vi "Experiment_pump_for_FR.vi"() -> ()   [LabVIEW 2016]
uses:
  <vilib>/Modbus/master/Create Master Instance (Serial).vi
  <vilib>/addons/control/pid/pid.llb/PID (DBL).vi
  <vilib>/Modbus/master/Modbus Master.lvclass
  database/database.lvlib
  <vilib>/Analysis/Matrix/NI_Matrix.lvlib
  <vilib>/addons/control/pid/NI_PID_pid.lvlib
  <vilib>/Analysis/Matrix/Numeric/Conversions/Array To Matrix - RA2.vi
panel:
  in  "单次时延(ms)":dbl
  in  "最大倍数":dbl
  out "阶跃测试输出":dbl
  out "倍数":dbl
  in  "TestId":string
  out "10s Timer":bool caption="结束"
  out "1s Timer":bool caption="结束"
  out "10ms Timer":bool caption="结束"
  in  "送风温度-流量":T1={"proportional gain (Kc)"=1.0, "integral time (Ti, min)"=40.0, "derivative time (Td, min)"=0.0}
  in  "设定流量":dbl format="%#.3f"
  in  "设定流量控制阀门-流量计读取":T1={"proportional gain (Kc)"=1.0, "integral time (Ti, min)"=40.0, "derivative time (Td, min)"=0.0}
  in  "Ctrl Strategy":u16
  in  "送风温度设定值":dbl format="%.2f"
  out "自动设定出风温度":dbl format="%.2f"
  in  "室内温度控制送风温度":T1={"proportional gain (Kc)"=1.0, "integral time (Ti, min)"=40.0, "derivative time (Td, min)"=0.0}
  in  "T setpoint":dbl format="%.2f"
  in  "根据阀门控制频率":T1={"proportional gain (Kc)"=1.0, "integral time (Ti, min)"=40.0, "derivative time (Td, min)"=0.0}
  in  "阀门开度设定值":dbl format="%.2f"
  in  "送风温度控制阀门":T1={"proportional gain (Kc)"=1.0, "integral time (Ti, min)"=40.0, "derivative time (Td, min)"=0.0}
  in  "电力控制水泵频率":T1={"proportional gain (Kc)"=1.0, "integral time (Ti, min)"=40.0, "derivative time (Td, min)"=0.0}
  in  "温差设定值":dbl format="%.2f"
  out "标记":dbl
  out "送回风温差":dbl
  in  "旁通压差设定值":dbl format="%.2f"
  out "阀门设定开度":dbl format="%.2f"
  in  "PID gains 2":T1={"proportional gain (Kc)"=1.0, "integral time (Ti, min)"=40.0, "derivative time (Td, min)"=0.0}
  in  "PID gains":T1={"proportional gain (Kc)"=1.0, "integral time (Ti, min)"=40.0, "derivative time (Td, min)"=0.0}
  in  "手动水泵频率设定":u16
  out "循环次数":i32
  out "水泵电耗设定值":dbl
  out "Data 2":string[][](array[string])
  in  "错误输入 16":errorcluster caption="错误输入"
  out "进水温度":sgl format="%.1f"
  out "频率":dbl caption="频  率" format="%.2f"
  out "error out 3":errorcluster
  in  "error in (no error)":errorcluster
  out "error out 2":errorcluster
  out "Data":string[][](array[string])
  out "布尔":bool
  in  "时间选择":bool
  out "波形图表":dynamicdata(graph)
  in  "手动加热百分比":u16 step=1
  out "error out 9":errorcluster
  in  "按时间查询":bool
  in  "多列列表框":i32(listbox)
  out "错误输出":errorcluster
  out "水泵转速":sgl format="%.2f"
  in  "出水温度设定":dbl step=1.0
  out "加热百分比":sgl format="%.2f"
  out "pv测量值":u16[](array[numeric]) caption="寄存器值"
  in  "阀设定开度":u16 step=1
  out "水泵设定频率":dbl step=1.0
  in  "error in (no error) 8":errorcluster caption="错误输入（无错误）"
  out "error out 6":errorcluster caption="错误输出"
  out "流量":dbl format="%.2f"
  out "进出口压力":dbl caption="进出口压差" format="%.2f"
  out "支管压差":dbl format="%.2f"
  out "回水温度":dbl format="%.1f"
  out "送风温度":dbl format="%.1f"
  out "回风温度":dbl format="%.1f"
  out "阀门开度":dbl format="%.2f"
  out "模拟量采集模块BD4141E 2":u16[](array[numeric]) caption="寄存器值"
  in  "error in (no error) 7":errorcluster caption="错误输入（无错误）"
  out "error out 5":errorcluster caption="错误输出"
  out "电流":dbl format="%#_4f"
  out "电压":dbl format="%.2f"
  out "水泵功率":dbl format="%.2f"
  in  "error in (no error) 3":errorcluster caption="错误输入（无错误）"
  out "通讯状态":bool
  in  "Stop":bool
  # "设  备   的  名  字"
  # "阶跃信号控制"
  # "设备的"
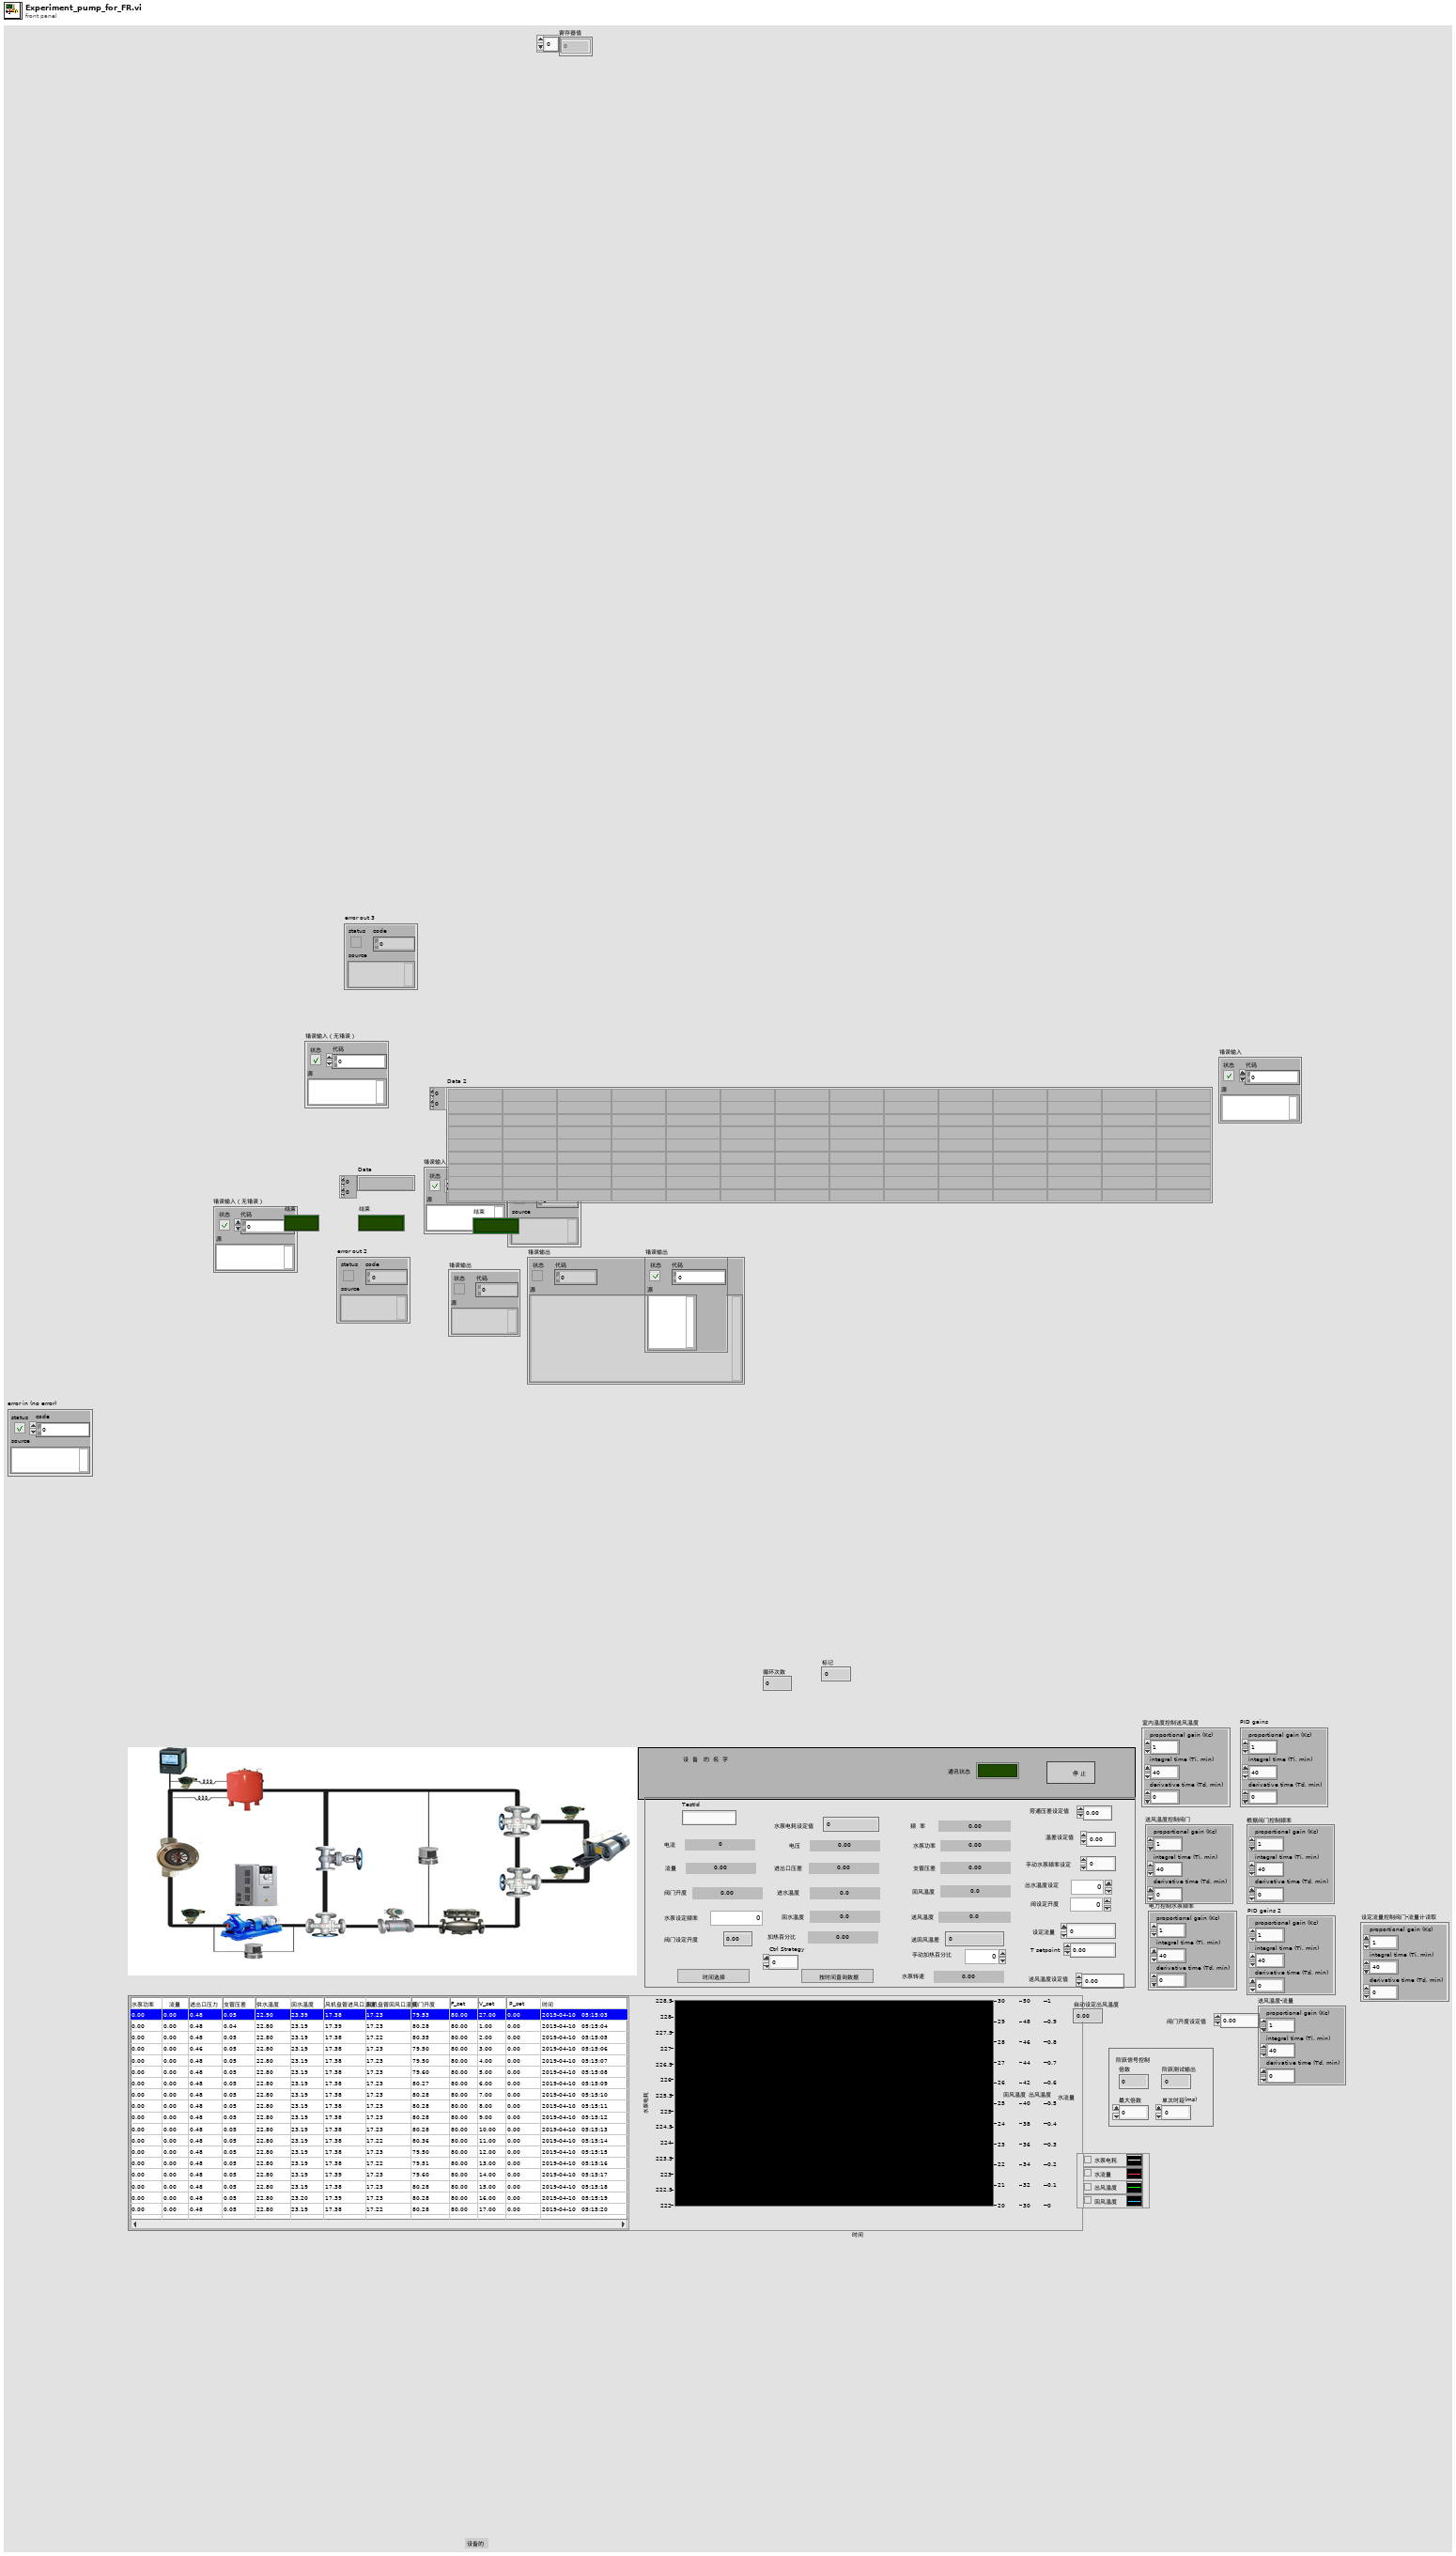
[diagram p1: front panel]
types:
  T1 = cluster{"proportional gain (Kc)":dbl, "integral time (Ti, min)":dbl, "derivative time (Td, min)":dbl}
  T2 = typedef "NI_Matrix.lvlib/RealMatrix.ctl" = dbl[][]
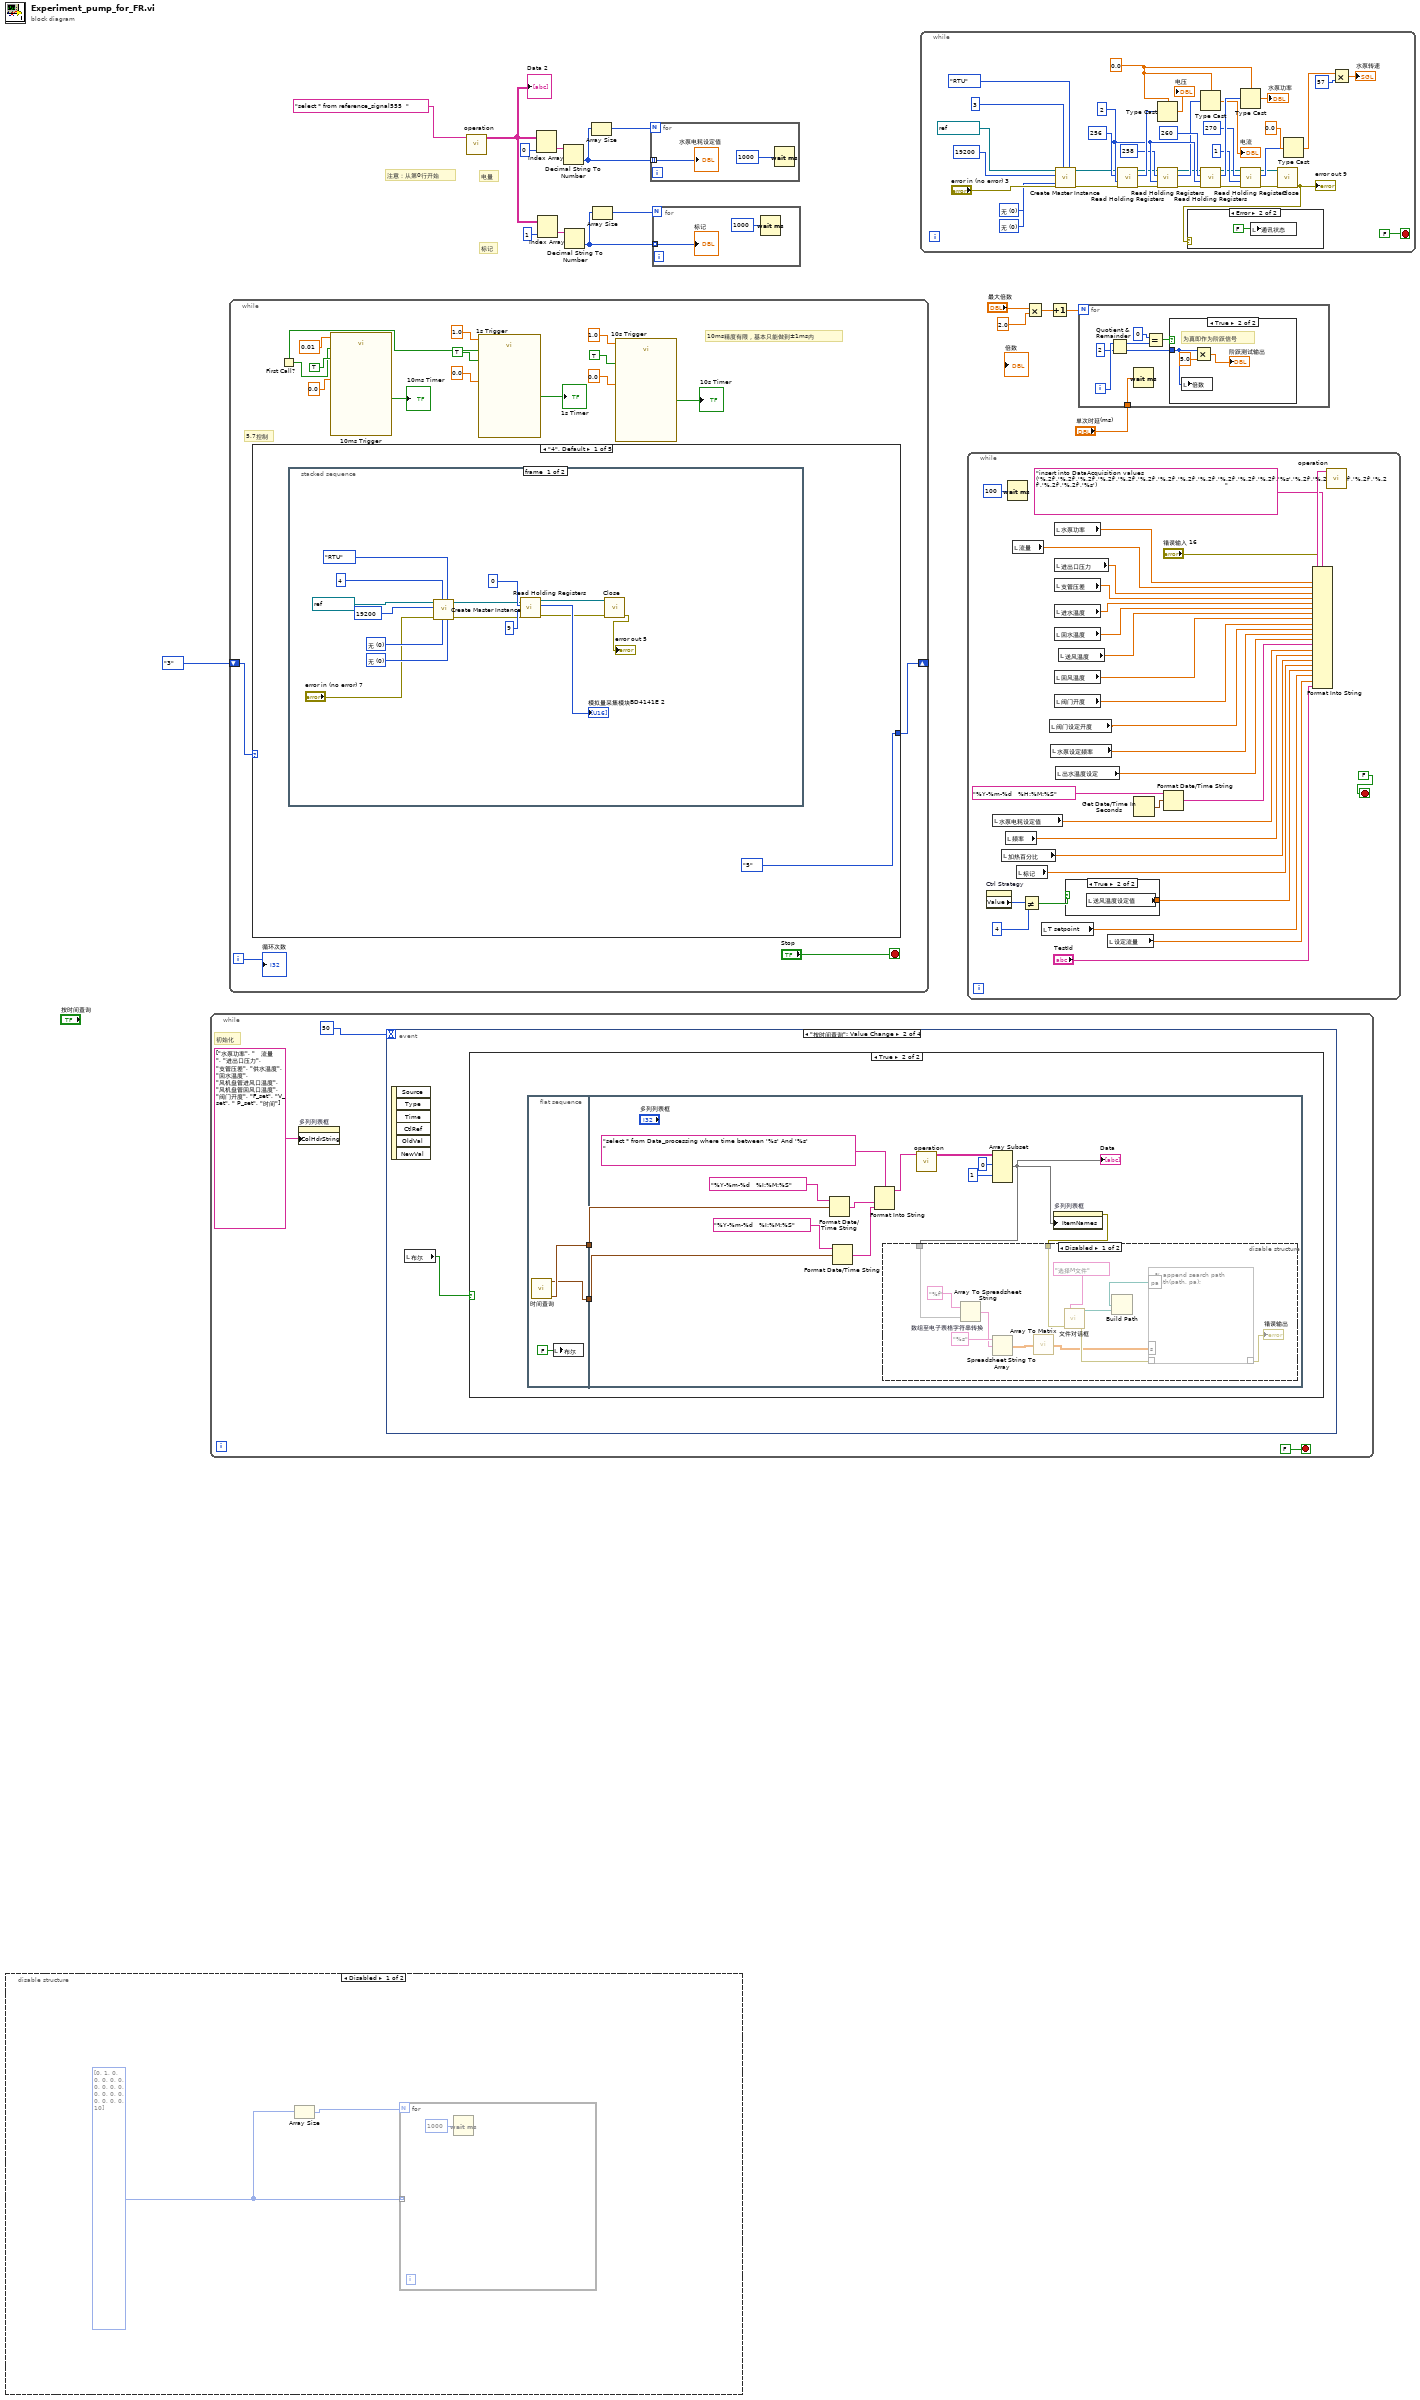
[diagram p0: block diagram]
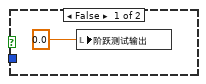
[diagram p2: hidden frame]
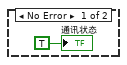
[diagram p3: hidden frame]
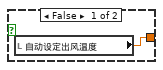
[diagram p4: hidden frame]
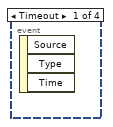
[diagram p6: hidden frame]
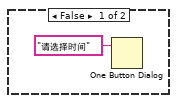
[diagram p7: hidden frame]
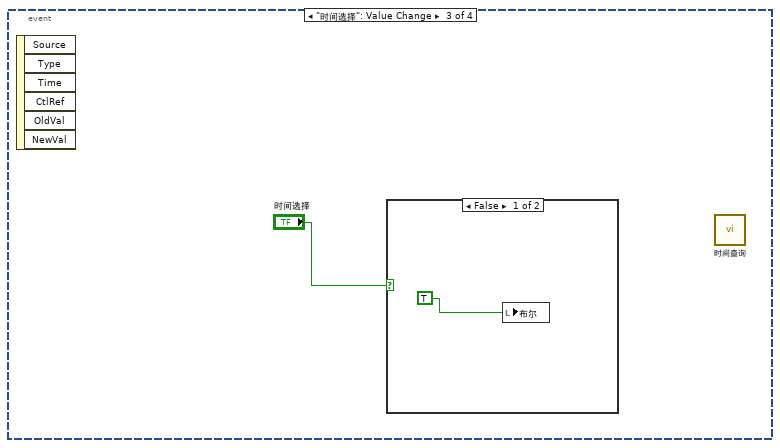
[diagram p9: hidden frame]
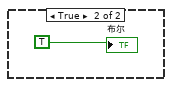
[diagram p10: hidden frame]
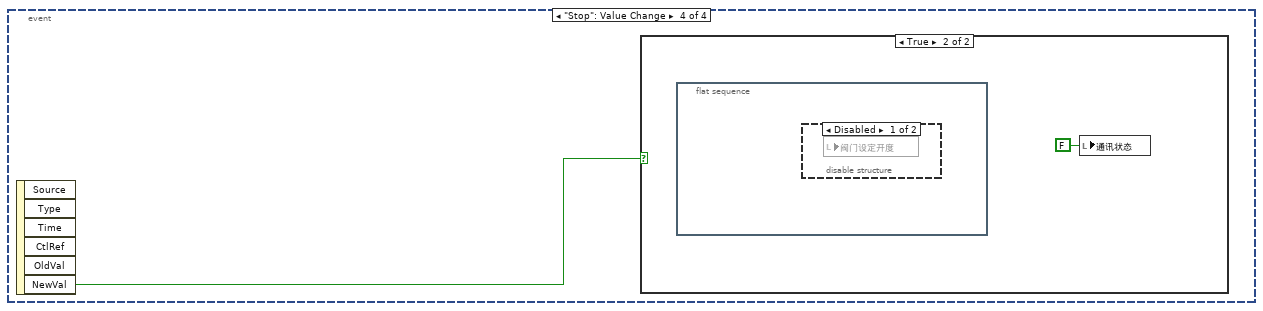
[diagram p11: hidden frame]
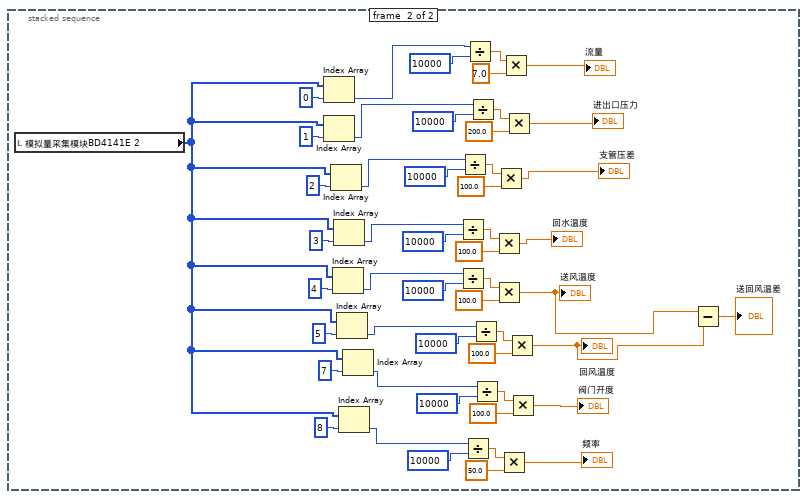
[diagram p14: hidden frame]
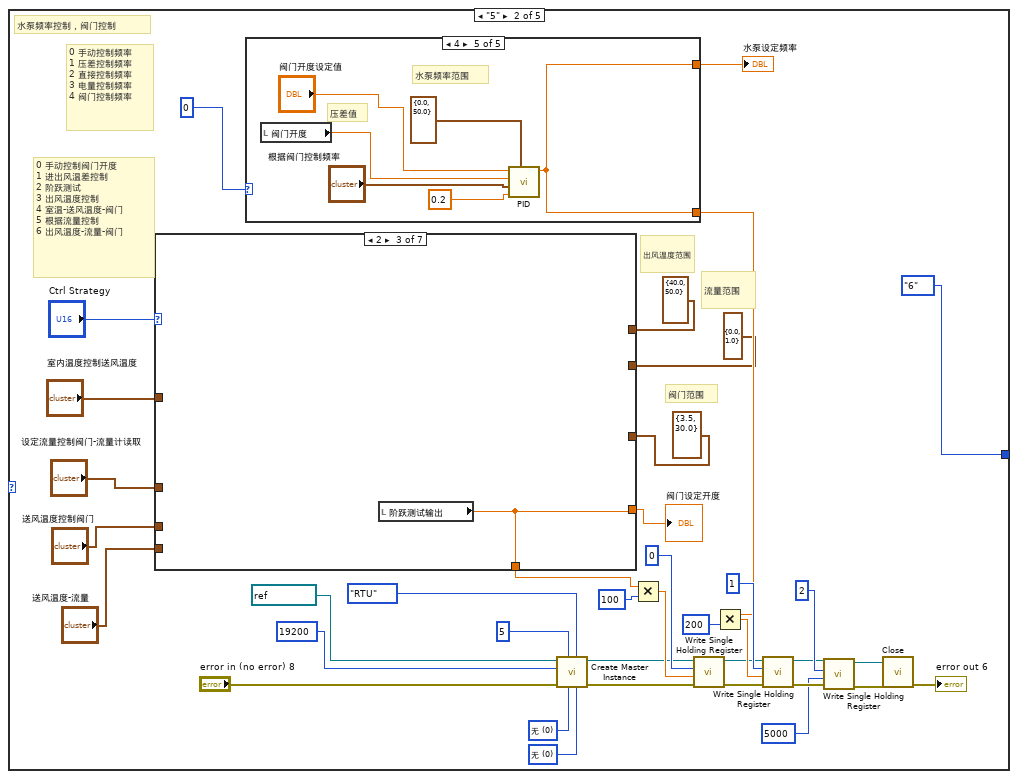
[diagram p15: hidden frame]
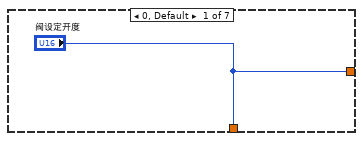
[diagram p16: hidden frame]
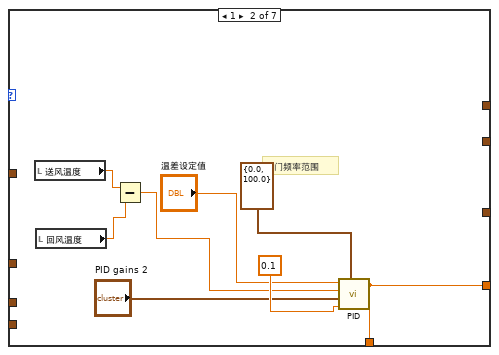
[diagram p17: hidden frame]
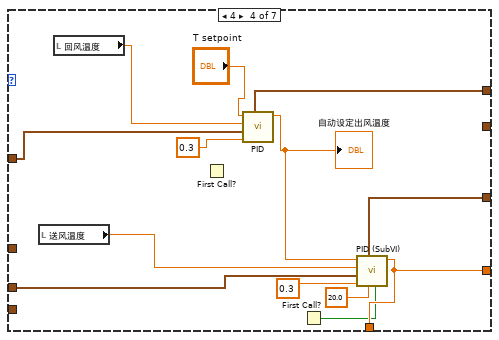
[diagram p18: hidden frame]
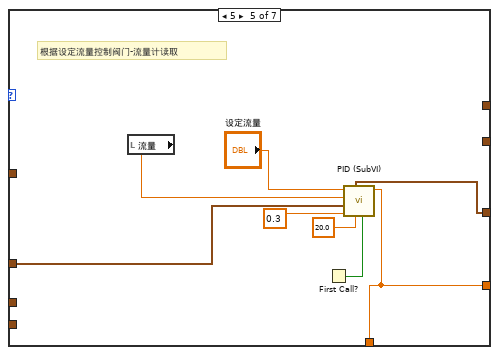
[diagram p19: hidden frame]
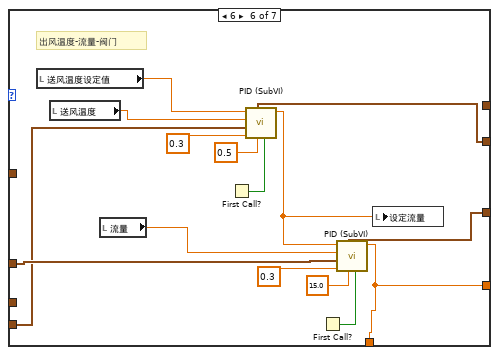
[diagram p20: hidden frame]
diagram:
  # "注意：从第0行开始"
  # "电量"
  # "标记"
  n1 = disable-structure shown="Disabled" {
    frame Disabled {
      w18 = i32[] [0, 1, 0, 0, 0, 0, 0, 0, 0, 0, 0, 0, 0, 0, 0, 0, 0, 0, 0, 10]
      n2 = Array Size(array=w18) -> (size(s)=w17:i32)
      n3 = for {
        N: w17 -> [_]
        tunnel: w18 -> [_] mode=indexing
        n4 = Wait (ms)(milliseconds to wait=u32 1000) -> ()  [unwired: 1 out]
      }
    }
    frame Enabled {
    }
  }
  n5 = while {
    stop <- FALSE stop-if-true
    # "初始化"
    n6 = property on="多列列表框" class="MCListbox (strict)"("ColHdrString"=string[] ["水泵功率", "   流量               ", "进出口压力", "支管压差", "供水温度", "回水温度", "风机盘管进风口温度", "风机盘管回风口温度", "阀门开度", "F_set", "V_set", " P_set", "时间"]) -> ()  [unwired: 2 in, 2 out]
    n7 = event shown="[1] \"按时间查询\": Value Change" {
      selector: _ -> [_ _ _ _]
      dyn-events: _ -> [_ _ _ _]
      timeout: 50 -> [_ _ _ _]
      event Timeout {
        n8 = event-data() -> ()  [unwired: 1 in, 3 out]
      }
      event "按时间查询": Value Change {
        n9 = event-data() -> ()  [unwired: 1 in, 6 out]
        n10 = local read "布尔"() -> (w23:bool)
        n11 = case shown="True" w23 {
          frame False {
            n12 = One Button Dialog(message="请选择时间" ("消息")) -> ()  [unwired: 1 in, 1 out]
          }
          frame True {
            n13 = flat-sequence {
              tunnel: [w28] -> w26
              tunnel: [w27] -> w25
              tunnel: w26 -> [w36]
              tunnel: w25 -> [w35]
              frame #0 {
                n14 = call "时间查询.vi"() -> ("时间标识 3"=w28:timestamp, "时间标识 4"=w27:timestamp)  [unwired: 8 in]
                n15 = local write "布尔"(FALSE ("布尔")) -> ()
              }
              frame #1 {
                n16 = Format Date/Time String(time format string (%c)="%Y-%m-%d   %I:%M:%S" ("时间格式字符串(%c)"), seconds (now)=w36) -> (date/time string=w40:string)  [unwired: 1 in]
                n17 = Format Date/Time String(time format string (%c)="%Y-%m-%d   %I:%M:%S" ("时间格式字符串(%c)"), seconds (now)=w35) -> (date/time string=w42:string)  [unwired: 1 in]
                n18 = Format Into String(format string="select * from Data_processing where time between '%s' And '%s'                                                                " ("格式字符串"), w40, w42) -> (resulting string=w37:string)  [unwired: 2 in, 1 out]
                n19 = call "operation.vi"("Command Text"=w37) -> ("Data"=w33:string[][])  [unwired: 9 in]
                n20 = Array Subset(array=w33, index (row)=0 ("index"), index (col)=1 ("index")) -> (w30:string[][])  [unwired: 2 in]
                "Data" <- w30
                n21 = property on="多列列表框" class="MCListbox (strict)"("ItemNames"=w30) -> (error out=w34:errorcluster)  [unwired: 2 in, 1 out]
                n22 = disable-structure shown="Disabled" {
                  disable-tunnel: w34 -> [w54 _]
                  disable-tunnel: w30 -> [w53 _]
                  frame Disabled {
                    n23 = Array To Spreadsheet String "数组至电子表格字符串转换"(array=w53, 3:"%f" ("格式字符串")) -> (spreadsheet string=w49:string)  [unwired: 1 in]
                    n24 = Spreadsheet String To Array(format string="%s" ("格式字符串"), spreadsheet string=w49) -> (array=w50:dbl[][])  [unwired: 2 in]
                    n25 = call-poly <vilib>:"Array To Matrix.vi"("Real 2D Array"=w50) -> ("Real Matrix"=w44:T2)
                    n26 = call "文件对话框"("prompt"="选择M文件", "error in"=w54) -> ("selected path"=w47:path, "error out"=w45:errorcluster)  [unwired: 10 in, 2 out]
                    n27 = Build Path(name or relative path=w47) -> (appended path=w46:path)  [unwired: 1 in]
                    n28 = script code="% append search path\npath(path, pa);"("??"=w45, "pa"=w46, "s"=w44) -> ("??"=→"错误输出":errorcluster)
                  }
                  frame Enabled {
                  }
                }
              }
            }
          }
        }
      }
      event "时间选择": Value Change {
        n29 = event-data() -> ()  [unwired: 1 in, 6 out]
        n30 = case shown="False" "时间选择" {
          frame False {
            n31 = local write "布尔"(TRUE) -> ()
          }
          frame True {
            "布尔" <- TRUE
          }
        }
        n32 = call "时间查询.vi"() -> ()  [unwired: 8 in, 2 out]
      }
      event "Stop": Value Change {
        n33 = event-data() -> ("NewVal"=w58:bool)  [unwired: 1 in, 5 out]
        n34 = case shown="True" w58 {
          frame False {
          }
          frame True {
            n35 = flat-sequence {
              frame #0 {
                n36 = disable-structure shown="Disabled" {
                  frame Disabled {
                    n37 = local read "阀门设定开度"() -> ()  [unwired: 1 in]
                  }
                  frame Enabled {
                  }
                }
              }
            }
            n38 = local write "通讯状态"(FALSE ("通讯状态")) -> ()
          }
        }
      }
    }
  }
  n39 = while {
    shift-right: [w75] -> _
    shift-left: enum16{"3", "4", "5", "6", "7", "8", "9", "10"}."3" -> [w76]
    i -> [w73]
    stop <- "Stop" stop-if-true
    # "10ms精度有限，基本只能做到±1ms内"
    # "5,7控制"
    n40 = case shown="\"4\", Default" w76 {
      tunnel: [enum16{"3", "4", "5", "6", "7", "8", "9", "10"}."5" enum16{"3", "4", "5", "6", "7", "8", "9", "10"}."6" enum16{"3", "4", "5", "6", "7", "8", "9", "10"}."7" enum16{"3", "4", "5", "6", "7", "8", "9", "10"}."8" enum16{"3", "4", "5", "6", "7", "8", "9", "10"}."3"] -> w75
      frame "4", Default {
        n41 = stacked-sequence {
          frame #0 {
            w86 = u16 0 items=["无", "XON/XOFF", "RTS/CTS", "XON/XOFF & RTS/CTS", "DTR/DSR", "XON/XOFF & DTR/DSR"] ("flow control (None)")
            w87 = u16 0 items=["无", "奇", "偶"] ("parity (Even)")
            n42 = call-poly <vilib>:"Create Master Instance.vi"("flow control (None)"=w86, "serial type"=enum16{"RTU", "ASCII"}."RTU", "parity (Even)"=w87, "unit ID"=u8 4, "error in (no error)"="error in (no error) 7", "baud rate (9600)"=u32 19200, "VISA resource name"=refnum<visa-resource-name> "COM4") -> ("error out"=w82:errorcluster, "serial master instance"=w79:refnum<class "Modbus Master.lvclass">)  [unwired: 3 in]
            n43 = call-dynamic "Read Holding Registers.vi"("error in (no error)"=w82, "number of holding registers"=u16 9, "starting address"=u16 0, "Modbus master in"=w79) -> ("error out"=w81:errorcluster, "register values"=→"模拟量采集模块BD4141E 2":u16[], "Modbus master out"=w78:refnum<class "Modbus Master.lvclass">)  [unwired: 5 in]
            n44 = call-dynamic "Close.vi"("error in (no error)"=w81, "Modbus master in"=w78) -> ("error out"=→"error out 5":errorcluster)  [unwired: 9 in]
          }
          frame #1 {
            n45 = local read "模拟量采集模块BD4141E 2"() -> (w102:u16[])
            n46 = Index Array(array=w102, index=0 ("索引")) -> (element=w135:u16)
            n47 = Index Array(array=w102, index=1 ("索引")) -> (element=w129:u16)
            n48 = Index Array(array=w102, index=2 ("索引")) -> (element=w123:u16)
            n49 = Index Array(array=w102, index=4 ("索引")) -> (element=w113:u16)
            n50 = Index Array(array=w102, index=3 ("索引")) -> (element=w119:u16)
            n51 = Index Array(array=w102, index=5 ("索引")) -> (element=w109:u16)
            n52 = Index Array(array=w102, index=8 ("索引")) -> (element=w98:u16)
            n53 = Index Array(array=w102, index=7 ("索引")) -> (element=w106:u16)
            n54 = Divide(x=w119, y=u16 10000) -> (x/y=w114:dbl)
            n55 = Divide(x=w113, y=u16 10000) -> (x/y=w115:dbl)
            n56 = Divide(x=w123, y=u16 10000) -> (x/y=w126:dbl)
            n57 = Divide(x=w98, y=u16 10000) -> (x/y=w101:dbl)
            n58 = Divide(x=w135, y=u16 10000) -> (x/y=w133:dbl)
            n59 = Divide(x=w129, y=u16 10000) -> (x/y=w128:dbl)
            n60 = Divide(x=w109, y=u16 10000) -> (x/y=w112:dbl)
            n61 = Divide(x=w106, y=u16 10000) -> (x/y=w105:dbl)
            n62 = Multiply(x=w114, y=100.0) -> (x*y=→"回水温度":dbl)
            n63 = Multiply(x=w115, y=100.0) -> (x*y=w96:dbl)
            "送风温度" <- w96
            n64 = Multiply(x=w126, y=100.0) -> (x*y=→"支管压差":dbl)
            n65 = Multiply(x=w101, y=50.0) -> (x*y=→"频率":dbl)
            n66 = Multiply(x=w133, y=7.0) -> (x*y=→"流量":dbl)
            n67 = Multiply(x=w128, y=200.0) -> (x*y=→"进出口压力":dbl)
            n68 = Multiply(x=w112, y=100.0) -> (x*y=w95:dbl)
            "回风温度" <- w95
            n69 = Multiply(x=w105, y=100.0) -> (x*y=→"阀门开度":dbl)
            n70 = Subtract(x=w96, y=w95) -> (x-y=→"送回风温差":dbl)
          }
        }
      }
      frame "5" {
        w174 = u16 0 items=["无", "XON/XOFF", "RTS/CTS", "XON/XOFF & RTS/CTS", "DTR/DSR", "XON/XOFF & DTR/DSR"] ("flow control (None)")
        w176 = u16 0 items=["无", "奇", "偶"] ("parity (Even)")
        # "流量范围"
        # "出风温度范围"
        # "阀门范围"
        # "0 手动控制阀门开度\n1 进出风温差控制\n2 阶跃测试\n3 出风温度控制\n4 室温-送风温度-阀门\n5 根据流量控制\n6 出风温度-流量-阀门"
        # "0 手动控制频率\n1 压差控制频率\n2 直接控制频率\n3 电量控制频率\n4 阀门控制频率"
        # "水泵频率控制，阀门控制"
        n71 = case shown="2" "Ctrl Strategy" {
          tunnel: ["阀设定开度" w182 w190 w200 w208 w223 w232] -> w161
          tunnel: ["阀设定开度" w182 w190 w200 w208 w223 w232] -> w160
          tunnel: "设定流量控制阀门-流量计读取" -> [_ _ _ _ w207 w221 _]
          tunnel: "室内温度控制送风温度" -> [_ _ _ w195 _ _ _]
          tunnel: cluster{"output high":dbl, "output low":dbl} {"output high"=3.5, "output low"=30.0} ("output range") -> [_ _ _ w194 w205 w222 _]
          tunnel: cluster{"output high":dbl, "output low":dbl} {"output high"=40.0, "output low"=50.0} ("output range") -> [_ _ _ w193 _ _ _]
          tunnel: "送风温度控制阀门" -> [_ _ _ w192 _ _ w227]
          tunnel: "送风温度-流量" -> [_ _ _ _ _ w215 _]
          tunnel: cluster{"output high":dbl, "output low":dbl} {"output high"=0.0, "output low"=1.0} ("output range") -> [_ _ _ _ _ w212 _]
          frame 0, Default {
          }
          frame 1 {
            # "阀门频率范围"
            n72 = local read "送风温度"() -> (w186:dbl)
            n73 = local read "回风温度"() -> (w185:dbl)
            n74 = Subtract(x=w186, y=w185) -> (x-y=w184:dbl)
            n75 = call-poly <vilib>:"PID.vi"("output range"=cluster{"output high":dbl, "output low":dbl} {"output high"=0.0, "output low"=100.0}, "dt (s)"=0.1, "PID gains"="PID gains 2", "process variable"=w184, "setpoint"="温差设定值") -> ("output"=w182:dbl)  [unwired: 5 in, 1 out]
          }
          frame 2 {
            n76 = local read "阶跃测试输出"() -> (w190:dbl)
          }
          frame 4 {
            n77 = local read "送风温度"() -> (w202:dbl)
            n78 = local read "回风温度"() -> (w197:dbl)
            n79 = First Call?() -> ()  [unwired: 1 out]
            n80 = call-poly <vilib>:"PID.vi"("output range"=w193, "dt (s)"=0.3, "PID gains"=w195, "process variable"=w197, "setpoint"="T setpoint") -> ("output"=w196:dbl)  [unwired: 5 in, 1 out]
            "自动设定出风温度" <- w196
            n81 = First Call?() -> (First Call?: T/F=w191:bool)
            n82 = call <userlib>:"PID (SubVI).vi"("reinitialize? (F)"=w191, "Initial Int"=20.0, "output range"=w194, "dt (s)"=0.3, "PID gains in"=w192, "Control variable"=w202, "SetPoint"=w196) -> ("output"=w200:dbl)  [unwired: 2 in, 2 out]
          }
          frame 5 {
            # "根据设定流量控制阀门-流量计读取"
            n83 = local read "流量"() -> (w210:dbl)
            n84 = First Call?() -> (First Call?: T/F=w204:bool)
            n85 = call <userlib>:"PID (SubVI).vi"("reinitialize? (F)"=w204, "Initial Int"=20.0, "output range"=w205, "dt (s)"=0.3, "PID gains in"=w207, "Control variable"=w210, "SetPoint"="设定流量") -> ("output"=w208:dbl)  [unwired: 2 in, 2 out]
          }
          frame 6 {
            # "出风温度-流量-阀门"
            n86 = local read "送风温度设定值"() -> (w214:dbl)
            n87 = local read "送风温度"() -> (w213:dbl)
            n88 = local read "流量"() -> (w216:dbl)
            n89 = First Call?() -> (First Call?: T/F=w220:bool)
            n90 = call <userlib>:"PID (SubVI).vi"("reinitialize? (F)"=w220, "Initial Int"=0.5, "output range"=w212, "dt (s)"=0.3, "PID gains in"=w215, "Control variable"=w213, "SetPoint"=w214) -> ("output"=w217:dbl)  [unwired: 2 in, 2 out]
            n91 = First Call?() -> (First Call?: T/F=w224:bool)
            n92 = call <userlib>:"PID (SubVI).vi"("reinitialize? (F)"=w224, "Initial Int"=15.0, "output range"=w222, "dt (s)"=0.3, "PID gains in"=w221, "Control variable"=w216, "SetPoint"=w217) -> ("output"=w223:dbl)  [unwired: 2 in, 2 out]
            n93 = local write "设定流量"(w217) -> ()
          }
          frame 3 {
            # "阀门范围"
            n94 = local read "送风温度"() -> (w234:dbl)
            n95 = property on="循环次数" class="DigNum (strict)"() -> ("Value"=w229:i32)  [unwired: 2 in, 2 out]
            n96 = Less?(x=w229, y=1) -> (x < y?=w228:bool)
            n97 = call <userlib>:"PID (SubVI).vi"("reinitialize? (F)"=w228, "Initial Int"=10.0, "output range"=cluster{"output high":dbl, "output low":dbl} {"output high"=3.5, "output low"=30.0}, "dt (s)"=0.3, "PID gains in"=w227, "Control variable"=w234, "SetPoint"="送风温度设定值") -> ("output"=w232:dbl)  [unwired: 2 in, 2 out]
          }
        }
        "阀门设定开度" <- w161
        n98 = case shown="4" u16 0 ("address") {
          tunnel: ["手动水泵频率设定" w238 w244 w246 w252] -> w162
          tunnel: ["手动水泵频率设定" w238 w244 w246 w252] -> w155
          frame 0, Default {
          }
          frame 1 {
            # "水泵频率范围"
            # "压差值"
            n99 = local read "支管压差"() -> (w240:dbl)
            n100 = call-poly <vilib>:"PID.vi"("output range"=cluster{"output high":dbl, "output low":dbl} {"output high"=0.0, "output low"=50.0}, "dt (s)"=0.1, "PID gains"="PID gains", "process variable"=w240, "setpoint"="旁通压差设定值") -> ("output"=w238:dbl)  [unwired: 5 in, 1 out]
          }
          frame 2 {
            n101 = property on="水泵电耗设定值" class="DigNum (strict)"() -> ("Value"=w244:dbl)  [unwired: 2 in, 2 out]
          }
          frame 3 {
            # "水泵频率范围"
            # "电量值"
            n102 = local read "水泵电耗设定值"() -> (w245:dbl)
            n103 = property on="水泵功率" class="DigNum (strict)"() -> ("Value"=w247:dbl)  [unwired: 2 in, 2 out]
            n104 = call-poly <vilib>:"PID.vi"("output range"=cluster{"output high":dbl, "output low":dbl} {"output high"=0.0, "output low"=50.0}, "dt (s)"=0.1, "PID gains"="电力控制水泵频率", "process variable"=w247, "setpoint"=w245) -> ("output"=w246:dbl)  [unwired: 5 in, 1 out]
          }
          frame 4 {
            # "水泵频率范围"
            # "压差值"
            n105 = local read "阀门开度"() -> (w251:dbl)
            n106 = call-poly <vilib>:"PID.vi"("output range"=cluster{"output high":dbl, "output low":dbl} {"output high"=0.0, "output low"=50.0}, "dt (s)"=0.2, "PID gains"="根据阀门控制频率", "process variable"=w251, "setpoint"="阀门开度设定值") -> ("output"=w252:dbl)  [unwired: 5 in, 1 out]
          }
        }
        "水泵设定频率" <- w155
        n107 = call-poly <vilib>:"Create Master Instance.vi"("flow control (None)"=w174, "serial type"=enum16{"RTU", "ASCII"}."RTU", "parity (Even)"=w176, "unit ID"=u8 5, "error in (no error)"="error in (no error) 8", "baud rate (9600)"=u32 19200, "VISA resource name"=refnum<visa-resource-name> "COM4") -> ("error out"=w169:errorcluster, "serial master instance"=w146:refnum<class "Modbus Master.lvclass">)  [unwired: 3 in]
        n108 = Multiply(x=w160, y=u16 100) -> (x*y=w167:dbl)
        n109 = call-dynamic "Write Single Holding Register.vi"("error in (no error)"=w169, "holding register value"=w167, "address"=u16 0, "Modbus master in"=w146) -> ("error out"=w166:errorcluster, "Modbus master out"=w145:refnum<class "Modbus Master.lvclass">)  [unwired: 6 in]
        n110 = Multiply(x=w162, y=u16 200) -> (x*y=w164:dbl)
        n111 = call-dynamic "Write Single Holding Register.vi"("error in (no error)"=w166, "holding register value"=w164, "address"=u16 1, "Modbus master in"=w145) -> ("error out"=w158:errorcluster, "Modbus master out"=w144:refnum<class "Modbus Master.lvclass">)  [unwired: 6 in]
        n112 = call-dynamic "Write Single Holding Register.vi"("error in (no error)"=w158, "holding register value"=u16 5000, "address"=u16 2, "Modbus master in"=w144) -> ("error out"=w159:errorcluster, "Modbus master out"=w143:refnum<class "Modbus Master.lvclass">)  [unwired: 6 in]
        n113 = call-dynamic "Close.vi"("error in (no error)"=w159, "Modbus master in"=w143) -> ("error out"=→"error out 6":errorcluster)  [unwired: 9 in]
      }
      frame "6" {
        n114 = flat-sequence {
          frame #0 {
            w268 = u16 0 items=["None", "XON/XOFF", "RTS/CTS", "XON/XOFF & RTS/CTS", "DTR/DSR", "XON/XOFF & DTR/DSR"] ("flow control (None)")
            w269 = u16 0 items=["None", "Odd", "Even"] ("parity (Even)")
            n115 = call-poly <vilib>:"Create Master Instance.vi"("flow control (None)"=w268, "serial type"=enum16{"RTU", "ASCII"}."RTU", "parity (Even)"=w269, "unit ID"=u8 6, "baud rate (9600)"=u32 19200, "VISA resource name"=refnum<visa-resource-name> "COM4") -> ("error out"=w262:errorcluster, "serial master instance"=w259:refnum<class "Modbus Master.lvclass">)  [unwired: 4 in]
            n116 = call-dynamic "Read Holding Registers.vi"("error in (no error)"=w262, "number of holding registers"=u16 3, "starting address"=u16 256, "Modbus master in"=w259) -> ("error out"=w260:errorcluster, "register values"=→"pv测量值":u16[], "Modbus master out"=w258:refnum<class "Modbus Master.lvclass">)  [unwired: 5 in]
            n117 = call-dynamic "Close.vi"("error in (no error)"=w260, "Modbus master in"=w258) -> ("error out"=→"error out 2":errorcluster)  [unwired: 9 in]
          }
          frame #1 {
            # "通讯地址6"
            n118 = local read "pv测量值"() -> (w278:u16[])
            n119 = Index Array(array=w278, index=0 ("索引")) -> (element=w277:u16)
            n120 = Index Array(array=w278, index=2 ("索引")) -> (element=w274:u16)
            n121 = Divide(x=w277, y=u16 10) -> (x/y=→"进水温度":dbl)
            n122 = Divide(x=w274, y=u16 10) -> (x/y=→"加热百分比":dbl)
          }
        }
      }
      frame "7" {
        w297 = u16 0 items=["None", "XON/XOFF", "RTS/CTS", "XON/XOFF & RTS/CTS", "DTR/DSR", "XON/XOFF & DTR/DSR"] ("flow control (None)")
        w298 = u16 0 items=["None", "Odd", "Even"] ("parity (Even)")
        # "温度控制"
        n123 = call-poly <vilib>:"Create Master Instance.vi"("flow control (None)"=w297, "serial type"=enum16{"RTU", "ASCII"}."RTU", "parity (Even)"=w298, "unit ID"=u8 6, "error in (no error)"="error in (no error)", "baud rate (9600)"=u32 19200, "VISA resource name"=refnum<visa-resource-name> "COM4") -> ("error out"=w290:errorcluster, "serial master instance"=w283:refnum<class "Modbus Master.lvclass">)  [unwired: 3 in]
        n124 = Multiply(x="出水温度设定", y=u16 10) -> (x*y=w286:dbl)
        n125 = call-dynamic "Write Single Holding Register.vi"("error in (no error)"=w290, "holding register value"=w286, "address"=u16 768 ("starting address"), "Modbus master in"=w283) -> ("error out"=w291:errorcluster, "Modbus master out"=w282:refnum<class "Modbus Master.lvclass">)  [unwired: 6 in]
        n126 = call-dynamic "Write Single Holding Register.vi"("error in (no error)"=w291, "holding register value"="手动加热百分比", "address"=u16 386 ("starting address"), "Modbus master in"=w282) -> ("error out"=w287:errorcluster, "Modbus master out"=w281:refnum<class "Modbus Master.lvclass">)  [unwired: 6 in]
        n127 = call-dynamic "Close.vi"("error in (no error)"=w287, "Modbus master in"=w281) -> ("error out"=→"error out 3":errorcluster)  [unwired: 9 in]
      }
      frame "8" {
        # "水泵电耗，水流量，出风温度，回风温度进行实时曲线变化显示"
        # "曲线显示"
        n128 = local read "送风温度"() -> (w304:dbl)
        n129 = local read "水泵功率"() -> (w306:dbl)
        n130 = local read "回风温度"() -> (w303:dbl)
        n131 = local read "流量"() -> (w305:dbl)
        n132 = Merge Signals(w306, w305, w304, w303) -> (→"波形图表":dynamicdata)
      }
    }
    n133 = First Call?() -> (First Call?: T/F=w66:bool)
    n134 = call "10ms Trigger"("Time Target (s)"=0.01, "Reset"=w66, "Auto Reset"=TRUE, "Set Start Time (s)"=0.0) -> ("Time has Elapsed"=→"10ms Timer":bool)  [unwired: 8 in, 7 out]
    n135 = call "1s Trigger"("Time Target (s)"=1.0, "Reset"=w66, "Auto Reset"=TRUE, "Set Start Time (s)"=0.0) -> ("Time has Elapsed"=→"1s Timer":bool)  [unwired: 8 in, 7 out]
    n136 = call "10s Trigger"("Time Target (s)"=1.0, "Auto Reset"=TRUE, "Set Start Time (s)"=0.0) -> ("Time has Elapsed"=→"10s Timer":bool)  [unwired: 9 in, 7 out]
    "循环次数" <- w73
  }
  n137 = call "operation.vi"("Command Text"="select * from reference_signal555  ") -> ("Data"=w8:string[][])  [unwired: 9 in]
  "Data 2" <- w8
  n138 = Index Array(array=w8, index (col)=0 ("disabled index (col)")) -> (element=w14:string[])  [unwired: 1 in]
  n139 = Index Array(array=w8, index (col)=1 ("disabled index (col)")) -> (element=w9:string[])  [unwired: 1 in]
  n140 = Decimal String To Number(string=w14) -> (number=w12:i32[])  [unwired: 2 in, 1 out]
  n141 = Decimal String To Number(string=w9) -> (number=w11:i32[])  [unwired: 2 in, 1 out]
  n142 = Array Size(array=w12) -> (size(s)=w13:i32)
  n143 = Array Size(array=w11) -> (size(s)=w10:i32)
  n144 = for {
    N: w13 -> [_]
    tunnel: w12 -> [w309] mode=indexing
    n145 = Wait (ms)(milliseconds to wait=u32 1000) -> ()  [unwired: 1 out]
    "水泵电耗设定值" <- w309
  }
  n146 = for {
    N: w10 -> [_]
    tunnel: w11 -> [w311] mode=indexing
    n147 = Wait (ms)(milliseconds to wait=u32 1000) -> ()  [unwired: 1 out]
    "标记" <- w311
  }
  n148 = while {
    stop <- FALSE stop-if-true
    w345 = sgl 0.0
    w332 = u16 2 ("number of holding registers")
    w323 = u16 0 items=["无", "XON/XOFF", "RTS/CTS", "XON/XOFF & RTS/CTS", "DTR/DSR", "XON/XOFF & DTR/DSR"] ("flow control (None)")
    w322 = u16 0 items=["无", "奇", "偶"] ("parity (Even)")
    n149 = call-poly <vilib>:"Create Master Instance.vi"("flow control (None)"=w323, "serial type"=enum16{"RTU", "ASCII"}."RTU", "parity (Even)"=w322, "unit ID"=u8 3, "error in (no error)"="error in (no error) 3", "baud rate (9600)"=u32 19200, "VISA resource name"=refnum<visa-resource-name> "COM5") -> ("error out"=w325:errorcluster, "serial master instance"=w316:refnum<class "Modbus Master.lvclass">)  [unwired: 3 in]
    n150 = call-dynamic "Read Holding Registers.vi"("error in (no error)"=w325, "number of holding registers"=w332, "starting address"=u16 256, "Modbus master in"=w316) -> ("error out"=w326:errorcluster, "register values"=w347:u16[], "Modbus master out"=w315:refnum<class "Modbus Master.lvclass">)  [unwired: 5 in]
    n151 = Type Cast(type=w345, x=w347) -> (*(type *) &x=→"电压":sgl)
    n152 = call-dynamic "Read Holding Registers.vi"("error in (no error)"=w326, "number of holding registers"=w332, "starting address"=u16 258, "Modbus master in"=w315) -> ("error out"=w327:errorcluster, "register values"=w329:u16[], "Modbus master out"=w314:refnum<class "Modbus Master.lvclass">)  [unwired: 5 in]
    n153 = Type Cast(type=w345, x=w329) -> (*(type *) &x=→"电流":sgl)
    n154 = call-dynamic "Read Holding Registers.vi"("error in (no error)"=w327, "number of holding registers"=w332, "starting address"=u16 260, "Modbus master in"=w314) -> ("error out"=w342:errorcluster, "register values"=w344:u16[], "Modbus master out"=w313:refnum<class "Modbus Master.lvclass">)  [unwired: 5 in]
    n155 = Type Cast(type=w345, x=w344) -> (*(type *) &x=→"水泵功率":sgl)
    n156 = call-dynamic "Read Holding Registers.vi"("error in (no error)"=w342, "number of holding registers"=u16 1, "starting address"=u16 270, "Modbus master in"=w313) -> ("error out"=w343:errorcluster, "register values"=w339:u16[], "Modbus master out"=w312:refnum<class "Modbus Master.lvclass">)  [unwired: 5 in]
    n157 = call-dynamic "Close.vi"("error in (no error)"=w343, "Modbus master in"=w312) -> ("error out"=w328:errorcluster)  [unwired: 9 in]
    "error out 9" <- w328
    n158 = case shown="Error" w328 {
      frame No Error {
        "通讯状态" <- TRUE
      }
      frame Error {
        n159 = local write "通讯状态"(FALSE) -> ()
      }
    }
    n160 = Type Cast(type=sgl 0.0, x=w339) -> (*(type *) &x=w341:sgl)
    n161 = Multiply(x=w341, y=57) -> (x*y=→"水泵转速":sgl)
  }
  n162 = while {
    stop <- FALSE stop-if-true
    n163 = property on="Ctrl Strategy" class="DigNum (strict)"() -> ("Value"=w355:u16)  [unwired: 2 in, 2 out]
    n164 = local read "水泵电耗设定值"() -> (w362:dbl)
    n165 = local read "加热百分比"() -> (w360:sgl)
    n166 = local read "频率"() -> (w361:dbl)
    n167 = Wait (ms)(milliseconds to wait=u32 100) -> ()  [unwired: 1 out]
    n168 = local read "流量"() -> (w371:dbl)
    n169 = local read "标记"() -> (w359:dbl)
    n170 = Not Equal?(x=w355, y=u16 4) -> (x != y?=w353:bool)
    n171 = local read "T setpoint"() -> (w356:dbl)
    n172 = local read "阀门设定开度"() -> (w363:dbl)
    n173 = local read "水泵设定频率"() -> (w380:dbl)
    n174 = local read "水泵功率"() -> (w370:dbl)
    n175 = local read "进出口压力"() -> (w372:dbl)
    n176 = local read "支管压差"() -> (w373:dbl)
    n177 = local read "进水温度"() -> (w374:sgl)
    n178 = local read "回水温度"() -> (w375:dbl)
    n179 = local read "回风温度"() -> (w378:dbl)
    n180 = local read "阀门开度"() -> (w379:dbl)
    n181 = local read "出水温度设定"() -> (w364:dbl)
    n182 = local read "送风温度"() -> (w376:dbl)
    n183 = case shown="True" w353 {
      tunnel: [w382 w383] -> w357
      frame False {
        n184 = local read "自动设定出风温度"() -> (w382:dbl)
      }
      frame True {
        n185 = local read "送风温度设定值"() -> (w383:dbl)
      }
    }
    n186 = local read "设定流量"() -> (w352:dbl)
    n187 = Get Date/Time In Seconds() -> (seconds since 1Jan1904=w366:timestamp)
    n188 = Format Date/Time String ("格式化日期/时间字符串")(time format string (%c)="%Y-%m-%d   %H:%M:%S" ("时间格式字符串(%c)"), seconds (now)=w366) -> (date/time string=w377:string)  [unwired: 1 in]
    n189 = Format Into String(format string="insert into DataAcquisition values ('%.2f','%.2f','%.2f','%.2f','%.2f','%.2f','%.2f','%.2f','%.2f','%.2f','%.2f','%.2f','%s','%.2f','%.2f','%.2f','%.2f','%.2f','%.2f','%.2f','%s')                                                                " ("格式字符串"), error in="错误输入 16", w370, w371, w372, w373, w374, w375, w376, w378, w379, w363, w380, w364, w377, w362, w361, w360, w359, w357, w356, w352, "TestId") -> (resulting string=w369:string)  [unwired: 1 in, 1 out]
    n190 = call "operation.vi"("Command Text"=w369) -> ()  [unwired: 9 in, 1 out]
  }
  n191 = Multiply(x="最大倍数", y=2.0) -> (x*y=w2:dbl)
  n192 = Increment(x=w2) -> (x+1=w1:dbl)
  n193 = for {
    N: w1 -> [_]
    tunnel: "单次时延(ms)" -> [w384]
    i -> [w390]
    n194 = Quotient & Remainder(x=w390, y=2) -> (x-y*floor(x/y)=w388:i32, floor(x/y)=w385:i32)
    n195 = Wait (ms)(milliseconds to wait=w384) -> ()  [unwired: 1 out]
    n196 = Equal?(x=0, y=w388) -> (x = y?=w386:bool)
    n197 = case shown="True" w386 {
      tunnel: w385 -> [_ w393]
      frame False {
        n198 = local write "阶跃测试输出"(0.0 ("实际开度")) -> ()
      }
      frame True {
        # "为真即作为阶跃信号"
        n199 = local write "倍数"(w393) -> ()
        n200 = Multiply(x=w393, y=5.0) -> (x*y=→"阶跃测试输出":dbl)
      }
    }
  }
